vi "Sdmi To Dkm.vi"(8 "error in (no error)":errorcluster, 10 "error":i32, 11 "sMiles":string) -> (0 "error out":i32, 1 "error out 2":errorcluster, 2 "dkm":dbl, 3 "sMiles out":string)   [LabVIEW 2023, in "POSCONV.lvlib"]
doc: "Converts string miles to double kilometres (One mile is 1.609344km)...\n\n\ndouble SdmiToDkm(char *sMiles, int *error);"
uses:
  POSCONV.lvlib
  C:/Users/J Gordon/Documents/Rail Tech/TV-HR/02 - Code/Modules/POSCONV/POSCONV.dll
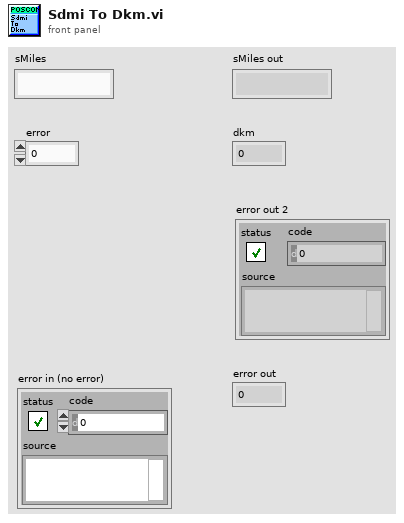
[diagram p1: front panel]
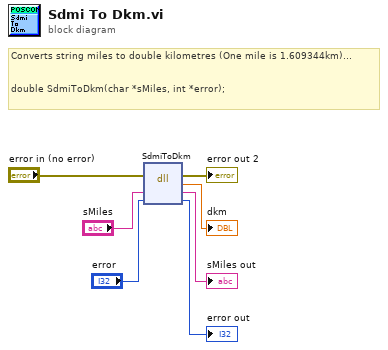
[diagram p0: block diagram]
diagram:
  # "Converts string miles to double kilometres (One mile is 1.609344km)...\n\n\ndouble SdmiToDkm(char *sMiles, int *error);"
  n1 = dll-call lib="C:/Users/J Gordon/Documents/Rail Tech/TV-HR/02 - Code/Modules/POSCONV/POSCONV.*" fn="SdmiToDkm"(error in="error in (no error)", "sMiles"="sMiles", "error"="error") -> (error out=→"error out 2":errorcluster, →"dkm":dbl, "sMiles"=→"sMiles out":string, "error"=→"error out":i32)  [unwired: 2 in, 1 out]
